vi "DCPowerInstrument_CallInitializeMeasurementLinkSessionWithCreateBehavior_RemoteSessionCreated.vi"(8 "error in":errorcluster) -> (0 "error out":errorcluster, 2 "result":string, 3 "pass":bool)   [LabVIEW 2020, in "MeasurementServerTests.lvlib"]
uses:
  MeasurementServerTests.lvlib
  Runtime/MeasurementLink Instrument/IInstrument/Initialize Session Behavior.ctl
  Runtime/MeasurementLink niDCPower/Instrument/Instrument.lvclass
  Runtime/MeasurementLink Instrument/IInstrument/IInstrument.lvclass
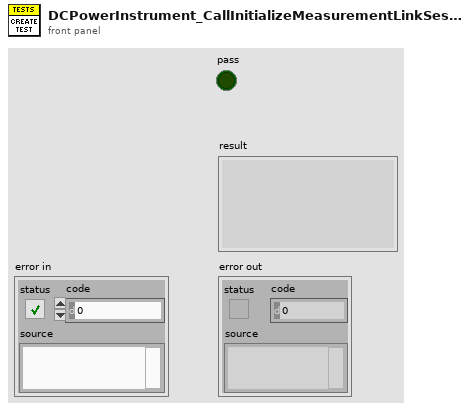
[diagram p1: front panel]
types:
  T1 = typedef "MeasurementLink Instrument.lvlib/IInstrument.lvclass/Remote Connection Options.ctl" = cluster{"session name":string, "address":string, "port":u32}
  T2 = typedef "MeasurementLink Instrument.lvlib/IInstrument.lvclass/Initialize Session Behavior.ctl" = enum16{"Create Session", "Attach Session"}
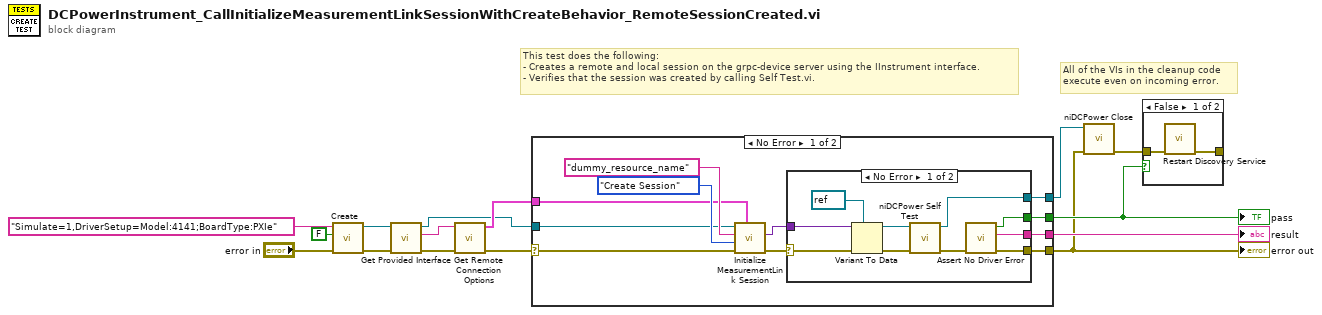
[diagram p0: block diagram]
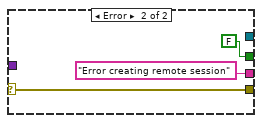
[diagram p2: hidden frame]
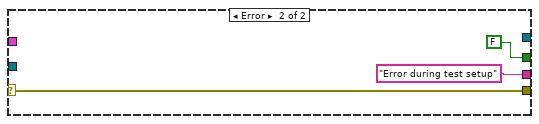
[diagram p3: hidden frame]
diagram:
  # "All of the VIs in the cleanup code\nexecute even on incoming error."
  # "This test does the following:\n- Creates a remote and local session on the grpc-device server using the IInstrument interface.\n- Verifies that the session was created by calling Self Test.vi."
  n1 = call "Create.vi"("error in"="error in", "reset"=FALSE, "option string"="Simulate=1,DriverSetup=Model:4141;BoardType:PXIe") -> ("error out"=w13:errorcluster, "instrument out"=w12:refnum<class "Instrument.lvclass">)  [unwired: 7 in]
  n2 = call-dynamic "Get Provided Interface.vi"("error in"=w13, "instrument in"=w12) -> ("error out"=w10:errorcluster, "provided interface"=w11:string, "instrument out"=w5:refnum<class "Instrument.lvclass">)  [unwired: 7 in]
  n3 = call "Get Remote Connection Options.vi"("error in"=w10, "provided interface"=w11) -> ("error out"=w7:errorcluster, "remote connection options"=w6:T1)  [unwired: 8 in]
  n4 = case shown="No Error" w7 {
    selector: w7 -> [w19 w40]
    tunnel: [w25 w40] -> w1
    tunnel: [w26 FALSE] -> w2
    tunnel: [w24 "Error during test setup" ("f")] -> w15
    tunnel: w6 -> [w18 _]
    tunnel: w5 -> [w17 _]
    tunnel: [w16 _] -> w4
    frame No Error {
      n5 = call-dynamic "Initialize MeasurementLink Session.vi"("remote connection options"=w18, "error in"=w19, "initialize session behavior"=Initialize_Session_Behavior."Create Session", "resource name"="dummy_resource_name", "instrument in"=w17) -> ("error out"=w22:errorcluster, "session out"=w23:variant)  [unwired: 4 in, 1 out]
      n6 = case shown="No Error" w22 {
        selector: w22 -> [w33 w38]
        tunnel: [w36 FALSE] -> w26
        tunnel: [w29 w38] -> w25
        tunnel: [w35 "Error creating remote session"] -> w24
        tunnel: w23 -> [w34 _]
        tunnel: [w28 _] -> w16
        frame No Error {
          n7 = Variant To Data(error in=w33, type=refnum<k15> refnum ("instrument handle"), Variant=w34) -> (data=w30:refnum<k15>, error out=w31:errorcluster)
          n8 = call <instrlib>:"niDCPower Self Test.vi"("error in (no error)"=w31, "instrument handle"=w30) -> ("error out"=w27:errorcluster, "instrument handle out"=w28:refnum<k15>)  [unwired: 6 in, 2 out]
          n9 = call "Assert No Driver Error.vi"("error in"=w27) -> ("error out"=w29:errorcluster, "result"=w35:string, "pass?"=w36:bool)  [unwired: 8 in]
        }
        frame Error {
        }
      }
    }
    frame Error {
    }
  }
  "error out" <- w1
  "pass" <- w2
  "result" <- w15
  n10 = call <instrlib>:"niDCPower Close.vi"("error in (no error)"=w1, "instrument handle"=w4) -> ("error out"=w3:errorcluster)  [unwired: 9 in]
  n11 = case shown="False" w2 {
    tunnel: w3 -> [w44 _]
    tunnel: [w43 _] -> _
    frame False {
      n12 = call "Restart Discovery Service.vi"("error in"=w44) -> ("error out"=w43:errorcluster)  [unwired: 10 in]
    }
    frame True {
    }
  }
